vi "Axis fgv.vi"(7 "Set":bool, 8 "error in (no error)":errorcluster, 11 "Axis":u16) -> (0 "error out":errorcluster, 3 "Axis out":u16)   [LabVIEW 2016]
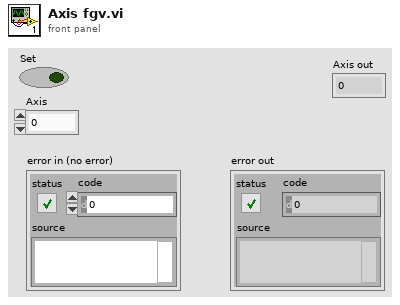
[diagram p1: front panel]
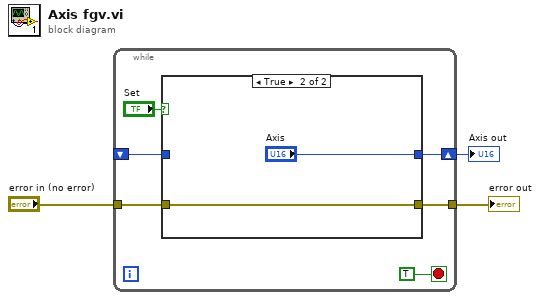
[diagram p0: block diagram]
diagram:
  n1 = while {
    shift-right: [w7] -> w3
    shift-left: _ -> [w6]
    tunnel: "error in (no error)" -> [w5]
    tunnel: [w4] -> w1
    stop <- TRUE stop-if-true
    n2 = case shown="True" "Set" {
      tunnel: [w11 "Axis"] -> w7
      tunnel: w6 -> [w11 _]
      tunnel: w5 -> [w10 w12]
      tunnel: [w10 w12] -> w4
      frame False {
      }
      frame True {
      }
    }
  }
  "Axis out" <- w3
  "error out" <- w1
